vi "Get Module Info.vi"(8 "error in":errorcluster, 11 "Module Detection in":refnum<class "Module Detection.lvclass">) -> (0 "error out":errorcluster, 2 "Module Info":T1[](array[typedef]) {"Product ID" format="%.0x"}, 3 "Module Detection out":refnum<class "Module Detection.lvclass">)   [LabVIEW 2015, in "RT Management.lvlib" / "Module Detection.lvclass"]
uses:
  Module Detection.lvclass
  Distributed Devices/Controls/DeviceInformation.ctl
  Distributed Devices/Device.lvclass
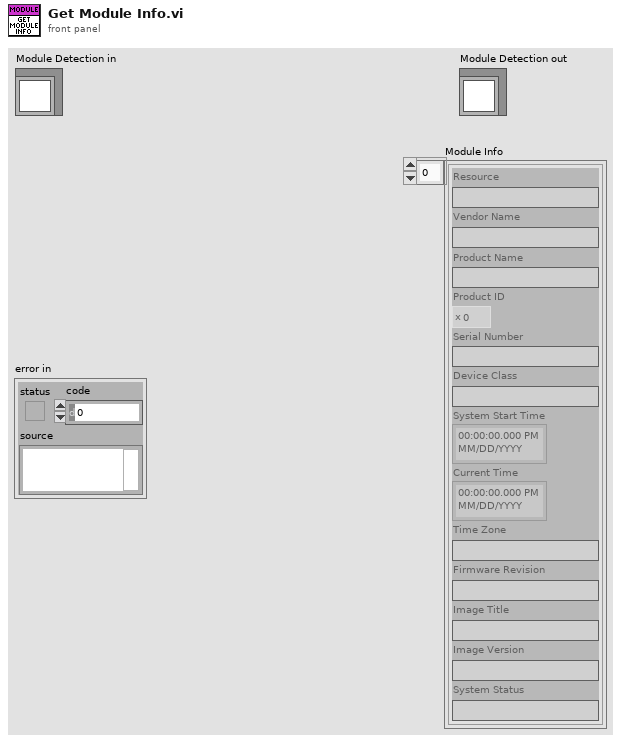
[diagram p1: front panel]
types:
  T1 = typedef "RT Management.lvlib/Device.lvclass/DeviceInformation.ctl" = cluster{"Resource":string, "Vendor Name":string, "Product Name":string, "Product ID":u32, "Serial Number":string, "Device Class":string, "System Start Time":timestamp, "Current Time":timestamp, "Time Zone":string, "Firmware Revision":string, "Image Title":string, "Image Version":string, "System Status":string}
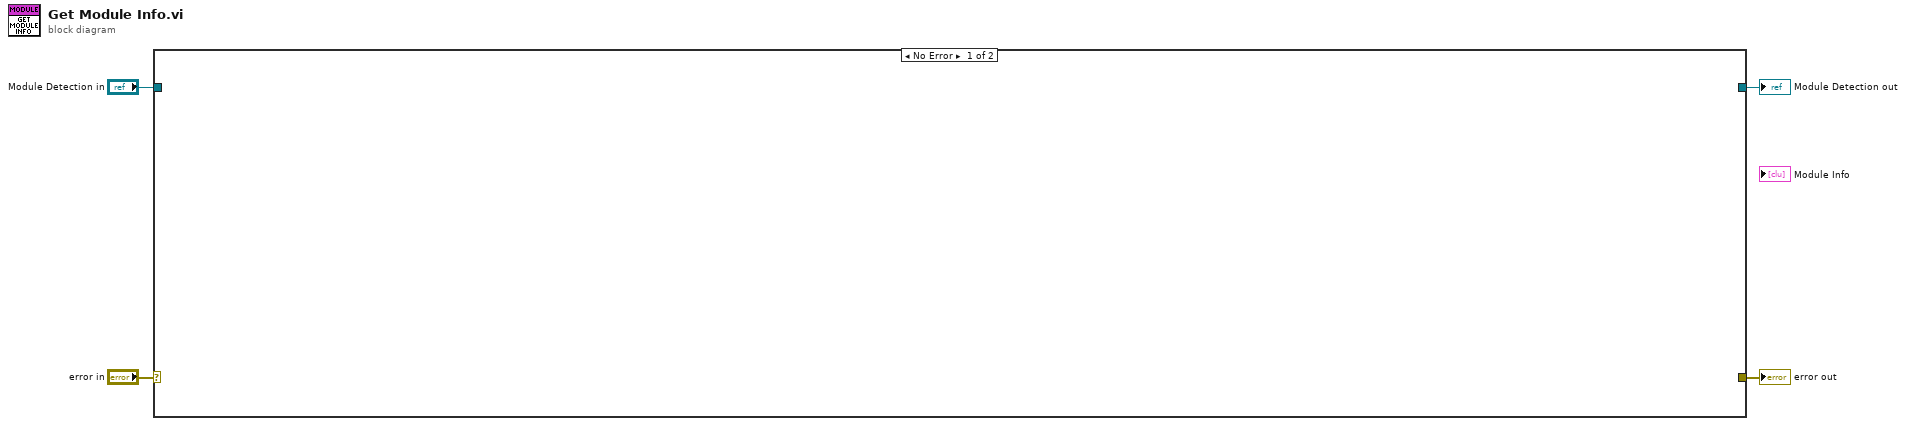
[diagram p0: block diagram]
diagram:
  n1 = case shown="No Error" "error in" {
    selector: "error in" -> [_ w6]
    tunnel: [_ w6] -> w3
    tunnel: [_ w5] -> w1
    tunnel: "Module Detection in" -> [_ w5]
    frame No Error {
    }
    frame Error {
    }
  }
  "error out" <- w3
  "Module Detection out" <- w1
